vi "(SubVI)_HR_Estimate.vi"(0 "Flow Signal":dbl[](array[numeric]), 5 "Samplin Freq":dbl) -> (4 "Heart Rate (bpm)":dbl, 6 "Heat Cycle (sec)":dbl)   [LabVIEW 2019]
uses:
  <vilib>/Analysis/4window.llb/Hanning Window (DBL).vi
  <vilib>/Analysis/2dsp.llb/Real FFT.vi
  <vilib>/Analysis/4window.llb/AllCosWindow (DBL).vi
  <vilib>/Analysis/NI_AALPro.lvlib
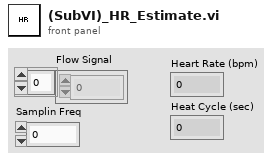
[diagram p1: front panel]
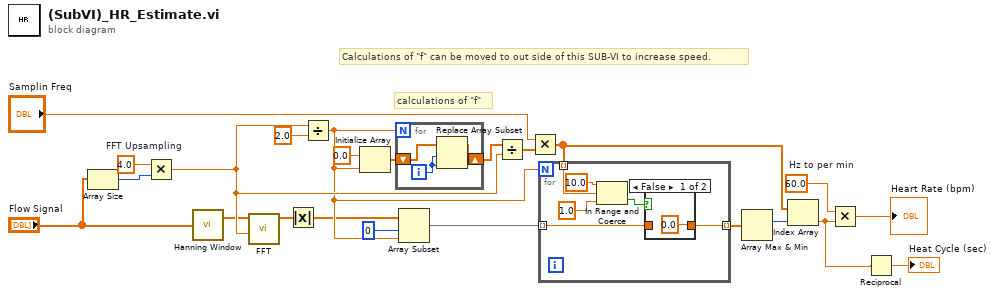
[diagram p0: block diagram]
diagram:
  w20 = 60.0  # Hz to per min
  w23 = 4.0  # FFT Upsampling
  # "calculations of \"f\""
  # "Calculations of \"f\" can be moved to out side of this SUB-VI to increase speed."
  n1 = Array Size(array="Flow Signal") -> (size(s)=w5:i32)
  n2 = Multiply(x=w23, y=w5) -> (x*y=w22:dbl)
  n3 = call-poly <vilib>:"Hanning Window.vi"("X"="Flow Signal") -> ("Windowed X"=w14:dbl[])  [unwired: 1 out]
  n4 = call-poly <vilib>:"FFT.vi"("FFT size"=w22, "X"=w14) -> ("FFT {X}"=w7:cdb[])  [unwired: 8 in, 1 out]
  n5 = Absolute Value(x=w7) -> (abs(x)=w12:dbl[])
  n6 = Divide(x=w22, y=2.0) -> (x/y=w15:dbl)
  n7 = Initialize Array(0.0 ("element"), w15) -> (w10:dbl[])
  n8 = for {
    N: w15 -> [_]
    shift-right: [w24] -> w6
    shift-left: w10 -> [w26]
    i -> [w25]
    n9 = Replace Array Subset(array=w26, new element=w25, index=w25) -> (w24:dbl[])
  }
  n10 = Array Subset(array=w12, index=0, length=w15) -> (w16:dbl[])
  n11 = Divide(x=w6, y=w22) -> (x/y=w11:dbl[])
  n12 = Multiply(x="Samplin Freq", y=w11) -> (x*y=w18:dbl[])
  n13 = for {
    N: w15 -> [_]
    tunnel: w18 -> [w30] mode=indexing
    tunnel: w16 -> [w28] mode=indexing
    tunnel: [w27] -> w17 mode=indexing
    n14 = In Range and Coerce(upper limit=10.0, x=w30, lower limit=1.0) -> (In Range?=w29:bool)  [unwired: 1 out]
    n15 = case shown="False" w29 {
      tunnel: w28 -> [_ w34]
      tunnel: [0.0 w34] -> w27
      frame False {
      }
      frame True {
      }
    }
  }
  n16 = Array Max & Min(array=w17) -> (max index (indices)=w19:i32)  [unwired: 3 out]
  n17 = Index Array(array=w18, index=w19) -> (element=w2:dbl)
  n18 = Multiply(x=w20, y=w2) -> (x*y=→"Heart Rate (bpm)":dbl)
  n19 = Reciprocal(x=w2) -> (1/x=→"Heat Cycle (sec)":dbl)
